vi "Couplingvi.vi"(5 "Motor":i32, 6 "Step per Sec":i32, 7 "Device Key":string, 8 "error in (no error)":errorcluster, 9 "LEFT/RIGHT COUPLE":bool, 10 "Device Address":i32, 11 ".NET Refnum in":refnum<k24>) -> (0 "error out":errorcluster, 1 "Device Address Out":i32, 2 "DeviceKey Out":string, 3 ".NET Refnum out":refnum<k24>, 4 "Direction":i32)   [LabVIEW 2021]
uses:
  C:/Program Files/New Focus/New Focus Picomotor Application/Samples/LabVIEW/Model 8742/LabVIEW 2009/CmdLib.dll
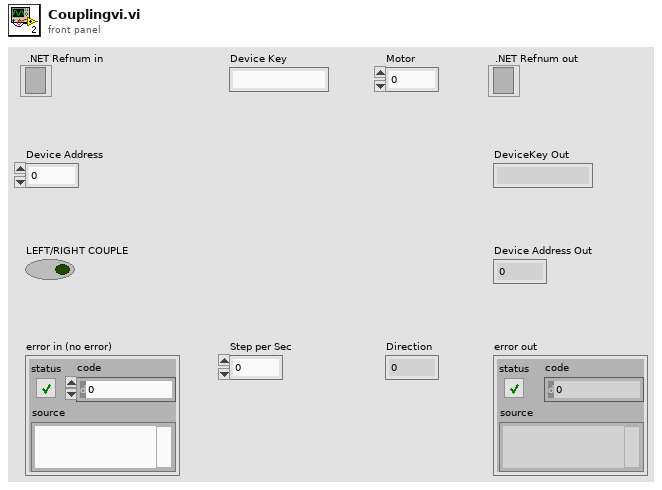
[diagram p1: front panel]
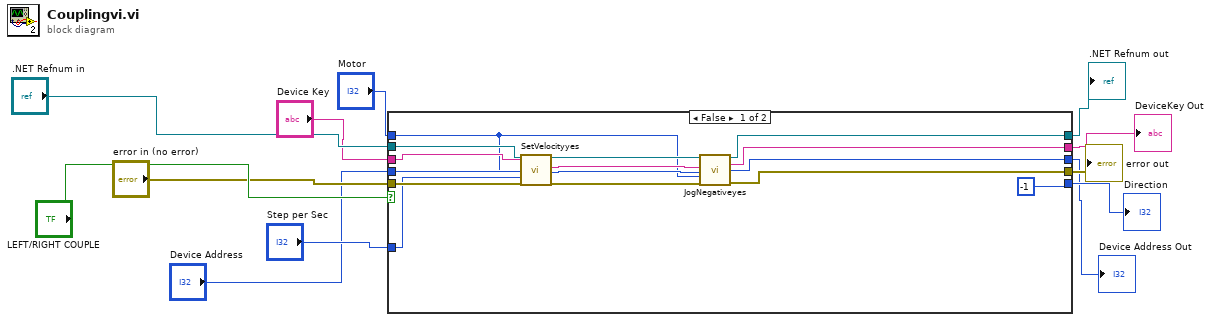
[diagram p0: block diagram]
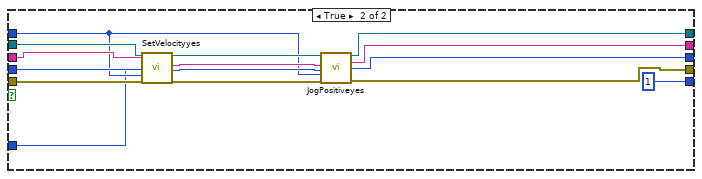
[diagram p2: hidden frame]
diagram:
  n1 = case shown="False" "LEFT/RIGHT COUPLE" {
    tunnel: "Motor" -> [w16 w31]
    tunnel: [w26 w42] -> w2
    tunnel: [w24 w41] -> w3
    tunnel: [w27 w40] -> w4
    tunnel: [w25 w39] -> w5
    tunnel: "Device Address" -> [w18 w33]
    tunnel: "Device Key" -> [w20 w35]
    tunnel: "error in (no error)" -> [w15 w30]
    tunnel: ".NET Refnum in" -> [w22 w37]
    tunnel: [-1 1] -> w11
    tunnel: "Step per Sec" -> [w13 w28]
    frame False {
      n2 = call "SetVelocityyes.vi"("CmdLib In"=w22, "DeviceKey In"=w20, "Device Address In"=w18, "Motor"=w16, "Steps Per Sec"=w13, "error in (no error)"=w15) -> ("CmdLib Out"=w21:refnum<k24>, "DeviceKey Out"=w19:string, "Device Address Out"=w17:i32, "error out"=w14:errorcluster)  [unwired: 10 in]
      n3 = call "JogNegativeyes.vi"("CmdLib In"=w21, "DeviceKey In"=w19, "Device Address In"=w17, "Motor"=w16, "error in (no error)"=w14) -> ("CmdLib Out"=w27:refnum<k24>, "DeviceKey Out"=w24:string, "Device Address Out"=w26:i32, "error out"=w25:errorcluster)  [unwired: 7 in]
    }
    frame True {
      n4 = call "SetVelocityyes.vi"("CmdLib In"=w37, "DeviceKey In"=w35, "Device Address In"=w33, "Motor"=w28, "Steps Per Sec"=w31, "error in (no error)"=w30) -> ("CmdLib Out"=w36:refnum<k24>, "DeviceKey Out"=w34:string, "Device Address Out"=w32:i32, "error out"=w29:errorcluster)  [unwired: 10 in]
      n5 = call "JogPositiveyes.vi"("CmdLib In"=w36, "DeviceKey In"=w34, "Device Address In"=w32, "Motor"=w31, "error in (no error)"=w29) -> ("CmdLib Out"=w40:refnum<k24>, "DeviceKey Out"=w41:string, "Device Address Out"=w42:i32, "error out"=w39:errorcluster)  [unwired: 7 in]
    }
  }
  "Direction" <- w11
  "error out" <- w5
  ".NET Refnum out" <- w4
  "DeviceKey Out" <- w3
  "Device Address Out" <- w2
